vi "I2C Read.vi"(9 "pdata":string, 10 "intAddress":u8, 11 "deviceID":u8) -> (1 "pdata out":string, 3 "function return":u32)   [LabVIEW 2018, in "Copy of Andor SDK.lvlib"]
doc: "EXPNETTYPE unsigned int WINAPI I2CRead(BYTE deviceID, BYTE intAddress, BYTE * pdata);"
uses:
  Copy of Andor SDK.lvlib
  <userlib>/Andor SDK/ATMCD32D.dll
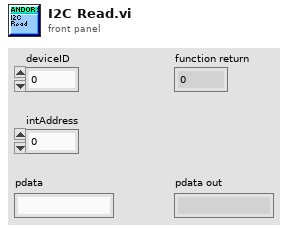
[diagram p1: front panel]
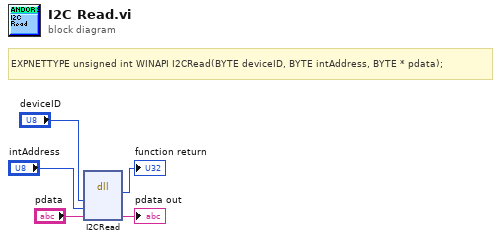
[diagram p0: block diagram]
diagram:
  # "EXPNETTYPE unsigned int WINAPI I2CRead(BYTE deviceID, BYTE intAddress, BYTE * pdata);"
  n1 = dll-call lib="C:/Program Files (x86)/National Instruments/LabVIEW 2018/user.lib/Andor SDK/ATMCD32D.*" fn="I2CRead"("deviceID"="deviceID", "intAddress"="intAddress", "pdata"="pdata") -> (→"function return":u32, "pdata"=→"pdata out":string)  [unwired: 5 in, 2 out]
